vi "Index.vi"(4 "case matching (sensitive)":T1=enum."system", 5 "default value":string, 6 "key":string, 7 "array in":T2) -> (1 "valid key":bool, 2 "value":string, 3 "duplicate array":T2)   [LabVIEW 2013, in "Tools_KeyedArray.lvlib"]
doc: "Returns the value of the element identified by <B>key</B>."
uses:
  Tools_KeyedArray.lvlib
  KeyedArray.ctl
  <vilib>/FTP/util/Case Matching.ctl
  <vilib>/FTP/NI_FTP.lvlib
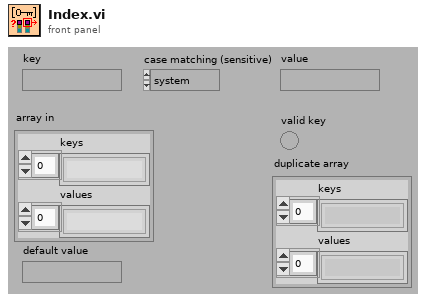
[diagram p1: front panel]
types:
  T1 = typedef "NI_FTP.lvlib/Case Matching.ctl" = enum16{"a != A", "a == A", "system"}
  T2 = typedef "Tools_KeyedArray.lvlib/KeyedArray.ctl" = cluster{"keys":string[], "values":string[]}
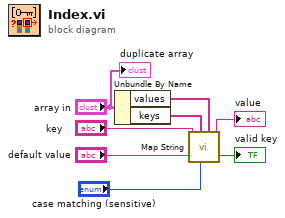
[diagram p0: block diagram]
diagram:
  n1 = Unbundle By Name("array in") -> ("values"=w4:string[], "keys"=w8:string[])
  n2 = call "Map String.vi"("default"="default value", "case matching (sensitive)"="case matching (sensitive)", "key"="key", "keys"=w8, "values"=w4) -> ("valid key"=→"valid key":bool, "value"=→"value":string)  [unwired: 1 out]
  "duplicate array" <- "array in"
